vi "Page Wrapper.vi"(8 "error in (no error)":errorcluster, 11 "Node Ptr":T1 format="%.0x") -> (0 "error out":errorcluster)   [LabVIEW 2020, in "Ballard ARINC 429 System Explorer.lvlib"]
uses:
  Ballard ARINC 429 System Explorer.lvlib
  Includes/Ballard ARINC 429 System Explorer.lvlibp/System Explorer/Interfaces/System Explorer Dispatcher/System Explorer Dispatcher.lvclass
  Includes/Ballard ARINC 429 System Explorer.lvlibp/System Explorer/Implementation/System Explorer Dispatcher/System Explorer Dispatcher.lvclass
  C:/git/ni/niveristand-communications-bus-template/Includes/Ballard ARINC 429 System Explorer.lvlibp/System Explorer/Implementation/System Explorer Dispatcher/System Explorer Dispatcher.lvclass
  C:/git/ni/niveristand-communications-bus-template/Includes/Ballard ARINC 429 System Explorer.lvlibp/System Explorer/Interfaces/System Explorer Dispatcher/System Explorer Dispatcher.lvclass
  <vilib>/NI VeriStand/Custom Device API/Custom Device Item Ref.ctl
  <vilib>/NI VeriStand/Custom Device API/Custom Device API.lvlib
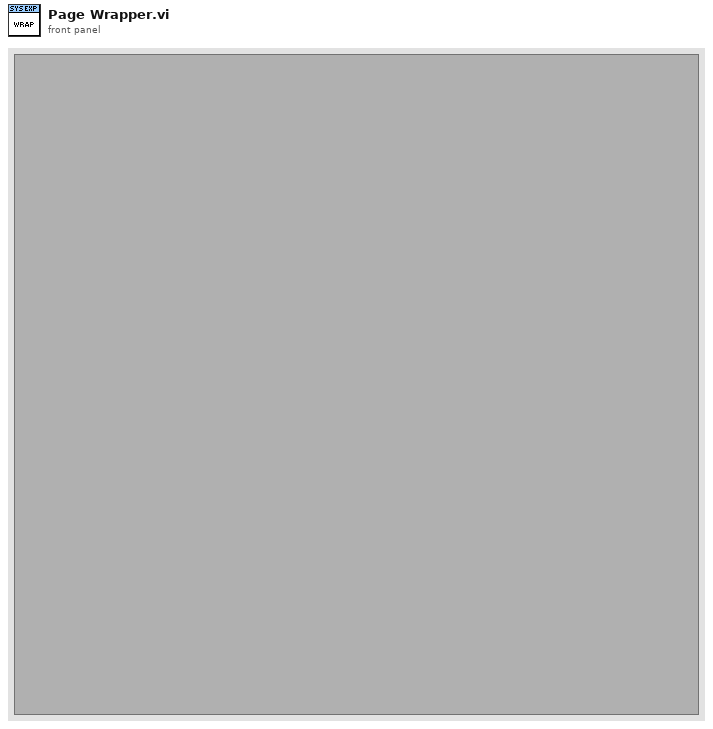
[diagram p1: front panel]
types:
  T1 = typedef "Custom Device API.lvlib/Custom Device Item Ref.ctl" = u64
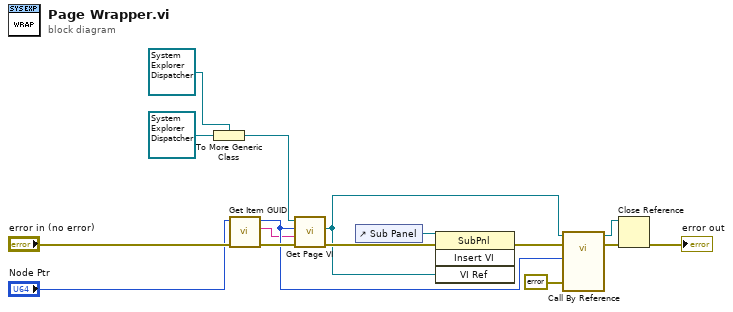
[diagram p0: block diagram]
diagram:
  n1 = To More Generic Class(target class=refnum<class "System Explorer Dispatcher.lvclass"> refnum ("Ballard ARINC 429 System Explorer.lvlibp:Interfaces.lvlib:System Explorer Dispatcher.lvclass"), reference=refnum<class "System Explorer Dispatcher.lvclass"> refnum ("Ballard ARINC 429 System Explorer.lvlibp:Implementation.lvlib:System Explorer Dispatcher.lvclass")) -> (generic class reference=w11:refnum<class "System Explorer Dispatcher.lvclass">)
  n2 = call "Get Item GUID.vi"("error in (no error)"="error in (no error)", "item in"="Node Ptr") -> ("error out"=w10:errorcluster, "guid"=w3:string, "item out"=w4:T1)  [unwired: 7 in]
  n3 = call-dynamic "Get Page VI.vi"("error in (no error)"=w10, "GUID"=w3, "Item Ref"=w4, "System Explorer Dispatcher in"=w11) -> ("error out"=w9:errorcluster, "page reference"=w8:refnum<vi>)  [unwired: 5 in, 1 out]
  n4 = control-ref of="Sub Panel"() -> (w13:refnum<vi>)
  n5 = invoke on="Invoke Node" class="SubPnl" method="Insert VI"(reference=w13, error in=w9, "VI Ref"=w8) -> (error out=w15:errorcluster)  [unwired: 1 in, 3 out]
  n6 = call-by-ref "?"(reference=w8, error in=w15, 8:"error in (no error)"=errorcluster {"status"=FALSE, "code"=0, "source"=""} ("error in (no error)"), "Node Ptr"=w4) -> (reference out=w6:refnum<vi>, error out=w14:errorcluster)  [unwired: 9 in, 1 out]
  n7 = Close Reference(reference=w6, error in (no error)=w14) -> (error out=→"error out":errorcluster)
